vi "getSignalPython.vi"() -> ()   [LabVIEW 2024]
uses:
  <vilib>/Analysis/Matrix/Datatypes/RealMatrix.ctl
  <vilib>/Analysis/Matrix/NI_Matrix.lvlib
panel:
  out "Waveform Graph":dbl[][](graph)
  out "submatrix":T1
  in  "stop":bool
  out "return value":T1
  in  "columnas":i32
  in  "filas":i32
  in  "Python version":string
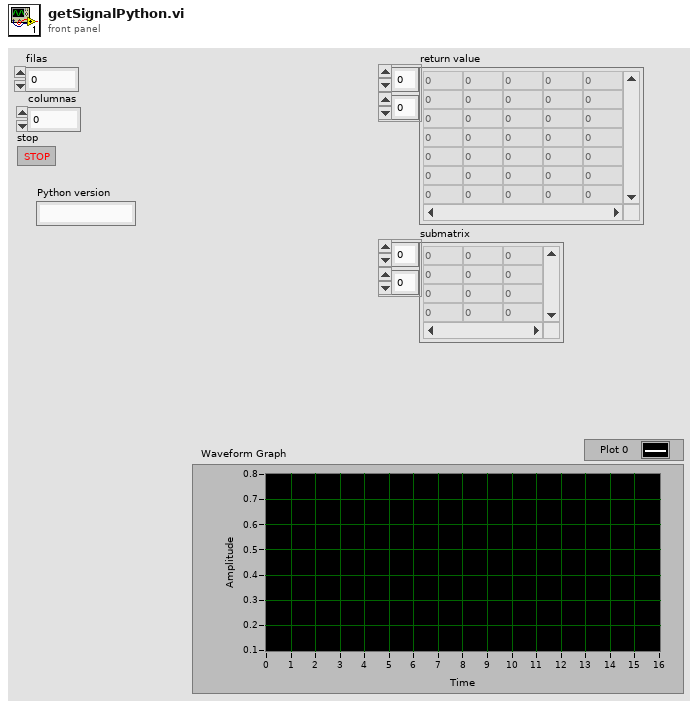
[diagram p1: front panel]
types:
  T1 = typedef "NI_Matrix.lvlib/RealMatrix.ctl" = dbl[][]
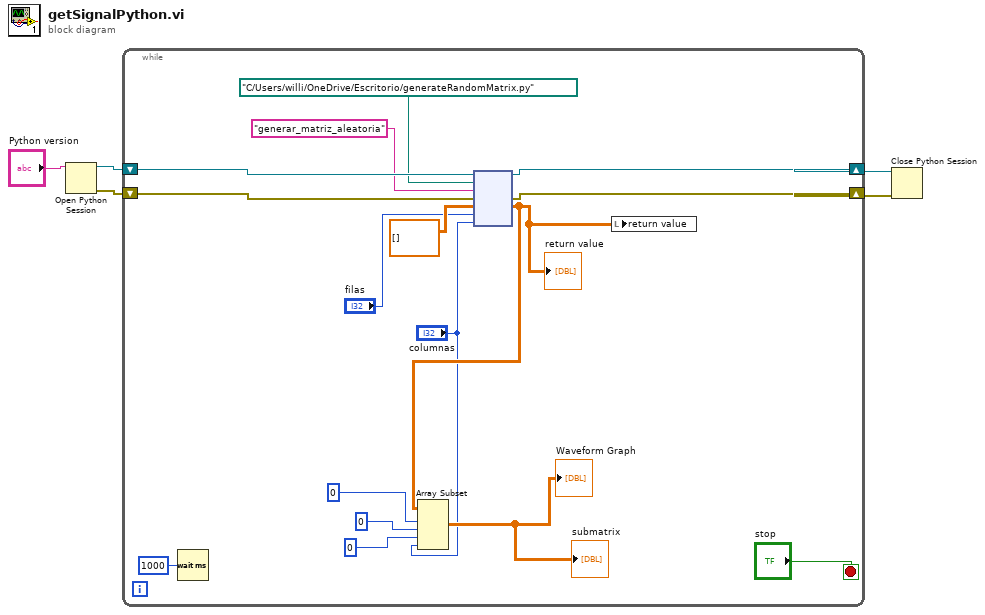
[diagram p0: block diagram]
diagram:
  n1 = Open Python Session(python version="Python version") -> (session out=w5:refnum<k35>, error out=w4:errorcluster)  [unwired: 2 in]
  n2 = while {
    shift-right: [w18] -> w2
    shift-left: w5 -> [w21]
    shift-right: [w19] -> w3
    shift-left: w4 -> [w20]
    stop <- "stop" stop-if-true
    n3 = Wait (ms)(milliseconds to wait=u32 1000) -> ()  [unwired: 1 out]
    n4 = node(w21, path "C:/Users/willi/OneDrive/Escritorio/generateRandomMatrix.py" ("module path"), "generar_matriz_aleatoria" ("function name"), w20, T1 [] ("Real Matrix"), "filas", "columnas") -> (w18:refnum<k35>, w19:errorcluster, w12:T1)  [unwired: 2 in, 2 out]
    "return value" <- w12
    n5 = Array Subset(array=w12, index (row)=0 ("row 1"), length (row)=0 ("column 1"), index (col)=0 ("column 1"), length (col)="columnas") -> (→"submatrix" →"Waveform Graph":T1)
    n6 = local write "return value"(w12) -> ()
  }
  n7 = Close Python Session(session in=w2, error in=w3) -> ()  [unwired: 1 out]
